vi "Wait.vi"(8 "error in (no error)":errorcluster, 11 "Event in":refnum<class "Event.lvclass">) -> (0 "error out":errorcluster, 1 "Timeout Occurred":bool=TRUE, 3 "Event out":refnum<class "Event.lvclass">)   [LabVIEW 2015, in "MDSplus.lvlib" / "Event.lvclass"]
doc: "Get data received as a raw buffer."
uses:
  Event.lvclass
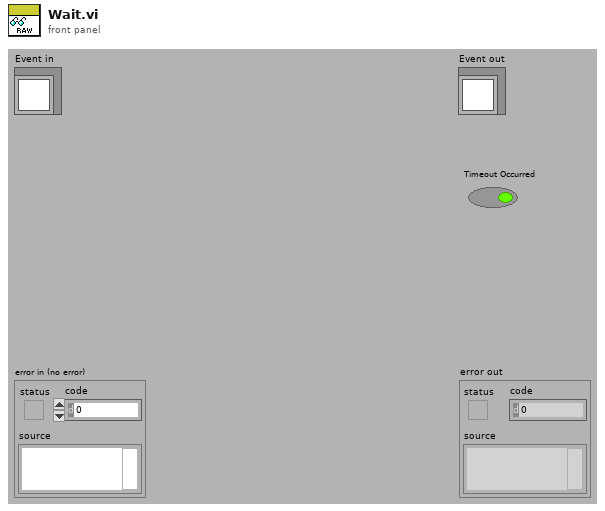
[diagram p1: front panel]
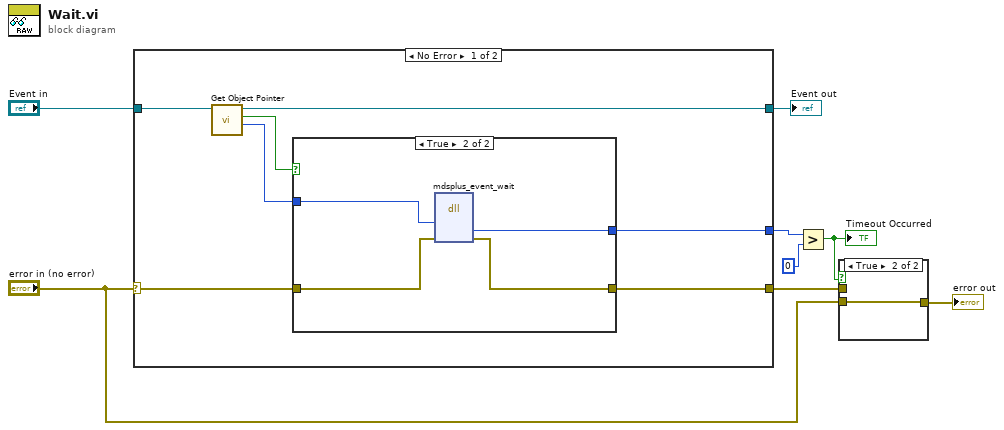
[diagram p0: block diagram]
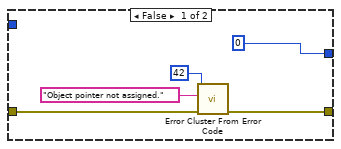
[diagram p3: hidden frame]
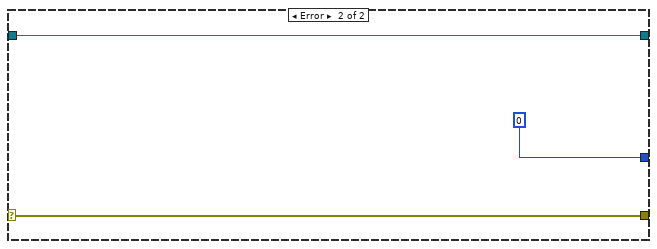
[diagram p4: hidden frame]
diagram:
  n1 = case shown="No Error" "error in (no error)" {
    selector: "error in (no error)" -> [w11 w27]
    tunnel: [w10 w27] -> w4
    tunnel: [w14 w26] -> w7
    tunnel: "Event in" -> [w15 w26]
    tunnel: [w9 0] -> w3
    frame No Error {
      n2 = call-dynamic "Get Object Pointer.vi"("Event in"=w15) -> ("Object Pointer"=w12:i64, "Assigned object pointer?"=w13:bool, "Event out"=w14:refnum<class "Event.lvclass">)  [unwired: 8 in]
      n3 = case shown="True" w13 {
        tunnel: w12 -> [_ w24]
        tunnel: w11 -> [w18 w23]
        tunnel: [w17 w22] -> w10
        tunnel: [0 ("error code (0)") w21] -> w9
        frame False {
          n4 = call <vilib>:"Error Cluster From Error Code.vi"("error in (no error)"=w18, "error message (\"\")"="Object pointer not assigned." ("error message (\"\")"), "error code (0)"=42) -> ("error out"=w17:errorcluster)  [unwired: 6 in]
        }
        frame True {
          n5 = dll-call lib="MDSobjectsLVShr" fn="mdsplus_event_wait"("lvEventPtr"=w24, "error"=w23) -> ("timeout"=w21:i32, "error"=w22:errorcluster)  [unwired: 6 in, 2 out]
        }
      }
    }
    frame Error {
    }
  }
  "Event out" <- w7
  n6 = Greater?(x=w3, y=0) -> (0:w6:bool)
  "Timeout Occurred" <- w6
  n7 = case shown="True" w6 {
    tunnel: "error in (no error)" -> [_ w29]
    tunnel: [w28 w29] -> w1
    tunnel: w4 -> [w28 _]
    frame False {
    }
    frame True {
    }
  }
  "error out" <- w1
